vi "Documentation.vi"   [LabVIEW 2019, in "Instrument.Framework-Template.lvclass"]
uses:
  Instrument.Framework-Template.lvclass
  9169cc93-ed84-4232-9f90-6ee16c7bb454.vi
  de41cf0e-ff2b-4a51-852c-55dbec0e345b.vi
  9169cc93-ed84-4232-9f90-6ee16c7bb454.vi/3bc1a7ce-2052-4bb6-955b-7b4bb15f1b3f.vi
  de41cf0e-ff2b-4a51-852c-55dbec0e345b.vi/21da6090-1418-40bf-b1d0-aaaa039838a5.vi
  9169cc93-ed84-4232-9f90-6ee16c7bb454.vi/3bc1a7ce-2052-4bb6-955b-7b4bb15f1b3f.vi/186c7484-df9a-4054-807c-655d760e15c8.vi
  SMOs/Instrument/API/Send and Receive.vi
  9169cc93-ed84-4232-9f90-6ee16c7bb454.vi/3bc1a7ce-2052-4bb6-955b-7b4bb15f1b3f.vi/d68663b6-9a59-49ac-8a3e-6c41418329a1.vi
  SMOs/Instrument/Private/Get Client Type.vi
  de41cf0e-ff2b-4a51-852c-55dbec0e345b.vi/21da6090-1418-40bf-b1d0-aaaa039838a5.vi/9c6ae891-6b7b-494d-b8a3-540145664cba.vi
  de41cf0e-ff2b-4a51-852c-55dbec0e345b.vi/21da6090-1418-40bf-b1d0-aaaa039838a5.vi/557a546d-74cb-4577-b055-fbd1aae73a04.vi
  9169cc93-ed84-4232-9f90-6ee16c7bb454.vi/3bc1a7ce-2052-4bb6-955b-7b4bb15f1b3f.vi/186c7484-df9a-4054-807c-655d760e15c8.vi/d1b53759-cdad-4b30-913c-d0af3a047282.vi
  9169cc93-ed84-4232-9f90-6ee16c7bb454.vi/3bc1a7ce-2052-4bb6-955b-7b4bb15f1b3f.vi/186c7484-df9a-4054-807c-655d760e15c8.vi/7fe9f392-2cd1-45ec-9a03-6ef05e8253b6.vi
  9169cc93-ed84-4232-9f90-6ee16c7bb454.vi/3bc1a7ce-2052-4bb6-955b-7b4bb15f1b3f.vi/d68663b6-9a59-49ac-8a3e-6c41418329a1.vi/8fac68c8-b375-4435-9af1-ae7d05afa959.vi
  9169cc93-ed84-4232-9f90-6ee16c7bb454.vi/3bc1a7ce-2052-4bb6-955b-7b4bb15f1b3f.vi/d68663b6-9a59-49ac-8a3e-6c41418329a1.vi/1362d31b-bfc4-4d78-893d-5589c90f5b2b.vi
  de41cf0e-ff2b-4a51-852c-55dbec0e345b.vi/21da6090-1418-40bf-b1d0-aaaa039838a5.vi/9c6ae891-6b7b-494d-b8a3-540145664cba.vi/19fa3c45-0d16-4bb0-b2ad-138c00be1b64.vi
  de41cf0e-ff2b-4a51-852c-55dbec0e345b.vi/21da6090-1418-40bf-b1d0-aaaa039838a5.vi/9c6ae891-6b7b-494d-b8a3-540145664cba.vi/55c769c2-5611-4ccb-aecc-8b538907d375.vi
  de41cf0e-ff2b-4a51-852c-55dbec0e345b.vi/21da6090-1418-40bf-b1d0-aaaa039838a5.vi/557a546d-74cb-4577-b055-fbd1aae73a04.vi/b0531fe4-9e29-4687-baa2-aadea3dcdf03.vi
  de41cf0e-ff2b-4a51-852c-55dbec0e345b.vi/21da6090-1418-40bf-b1d0-aaaa039838a5.vi/557a546d-74cb-4577-b055-fbd1aae73a04.vi/d5c1aeff-1834-4139-868c-d1c2b7ad11df.vi
  9169cc93-ed84-4232-9f90-6ee16c7bb454.vi/3bc1a7ce-2052-4bb6-955b-7b4bb15f1b3f.vi/d68663b6-9a59-49ac-8a3e-6c41418329a1.vi/8fac68c8-b375-4435-9af1-ae7d05afa959.vi/29d737dc-f0a6-4278-8ea1-10f2043af5e9.vi
  9169cc93-ed84-4232-9f90-6ee16c7bb454.vi/3bc1a7ce-2052-4bb6-955b-7b4bb15f1b3f.vi/d68663b6-9a59-49ac-8a3e-6c41418329a1.vi/8fac68c8-b375-4435-9af1-ae7d05afa959.vi/10a74567-eb18-4897-8559-1a35f16d5028.vi
  de41cf0e-ff2b-4a51-852c-55dbec0e345b.vi/21da6090-1418-40bf-b1d0-aaaa039838a5.vi/557a546d-74cb-4577-b055-fbd1aae73a04.vi/b0531fe4-9e29-4687-baa2-aadea3dcdf03.vi/aeda4fc1-3546-460b-8fa5-afdc0bea1e87.vi
  de41cf0e-ff2b-4a51-852c-55dbec0e345b.vi/21da6090-1418-40bf-b1d0-aaaa039838a5.vi/557a546d-74cb-4577-b055-fbd1aae73a04.vi/b0531fe4-9e29-4687-baa2-aadea3dcdf03.vi/ed5f9993-61e6-48eb-895f-b725d41d8077.vi
  SMOs/Instrument/Private/Get RC Connection Status.vi
  SMOs/Instrument/API/Enum to String.vi
  SMOs/RemoteControl/API/Send and Receive.vi
  <vilib>/Utility/Data Type/Get Type Information.vi
  <vilib>/JDP Science/JSONtext/JSON text to Variant.vi
  SMOs/Instrument/API/Instrument.GetPublicEvents.vi
  <vilib>/JDP Science/JSONtext/Variant to JSON Text.vi
  <vilib>/National Instruments/GUID Generator/Guid Generator.vi
  SMOs/Instrument/Private/Instrument.MessageFromProcess.EventStructure.vi
  SMOs/Instrument/Instrument.lvclass
  <vilib>/JKI/JKI SMO/SMO/SMO.lvclass
  Typedefs/Instrument.Framework-Template.Commands--Enum.ctl
  Typedefs/Instrument.Framework-Template.getAll--Cluster.ctl
  Typedefs/Instrument.Framework-Template.Configuration--Cluster.ctl
  <vilib>/JDP Science/JSONtext/LVClass Serializer/JSONtext LVClass Serializer.lvclass
  Instrument UI.Framework-Template/Instrument UI.Framework-Template.lvclass
  Instrument UI.Framework-Template/Instrument UI.Framework-Template.UI--Cluster.ctl
  SMOs/Instrument UI/Instrument UI.lvclass
  <vilib>/JKI/JKI SMO/SMO.UI/SMO.UI.lvclass
  C:/Program Files (x86)/National Instruments/LabVIEW 2019/vi.lib/JKI/JKI SMO/SMO/SMO.lvclass
  C:/Users/patrick/Documents/GitHub/Instrument-Framework/lvsrc/SMOs/Instrument/Instrument.lvclass
  C:/Users/patrick/Documents/GitHub/Instrument-Framework/lvsrc/SMOs/Instrument UI/Instrument UI.lvclass
  C:/Program Files (x86)/National Instruments/LabVIEW 2019/vi.lib/JKI/JKI SMO/SMO.UI/SMO.UI.lvclass
types:
  T1 = typedef "Instrument.Framework-Template.lvclass/Instrument.Framework-Template.Configuration--Cluster.ctl" = cluster{"Example Setting 1":dbl, "Example Setting 2":dbl, "Example Setting 3":string}
  T2 = typedef "Instrument.Framework-Template.lvclass/Instrument.Framework-Template.getAll--Cluster.ctl" = cluster{"Levy 1":dbl, "Logger SMO":dbl, "SMO Boolean":bool, "SMO String":string}
  T3 = typedef "Instrument.Framework-Template.lvclass/Instrument.Framework-Template.Commands--Enum.ctl" = enum16{"Do Something"}
  T4 = typedef "Instrument UI.Framework-Template.lvclass/Instrument UI.Framework-Template.UI--Cluster.ctl" = cluster{"Parameter":dbl, "Parameter 2":string}
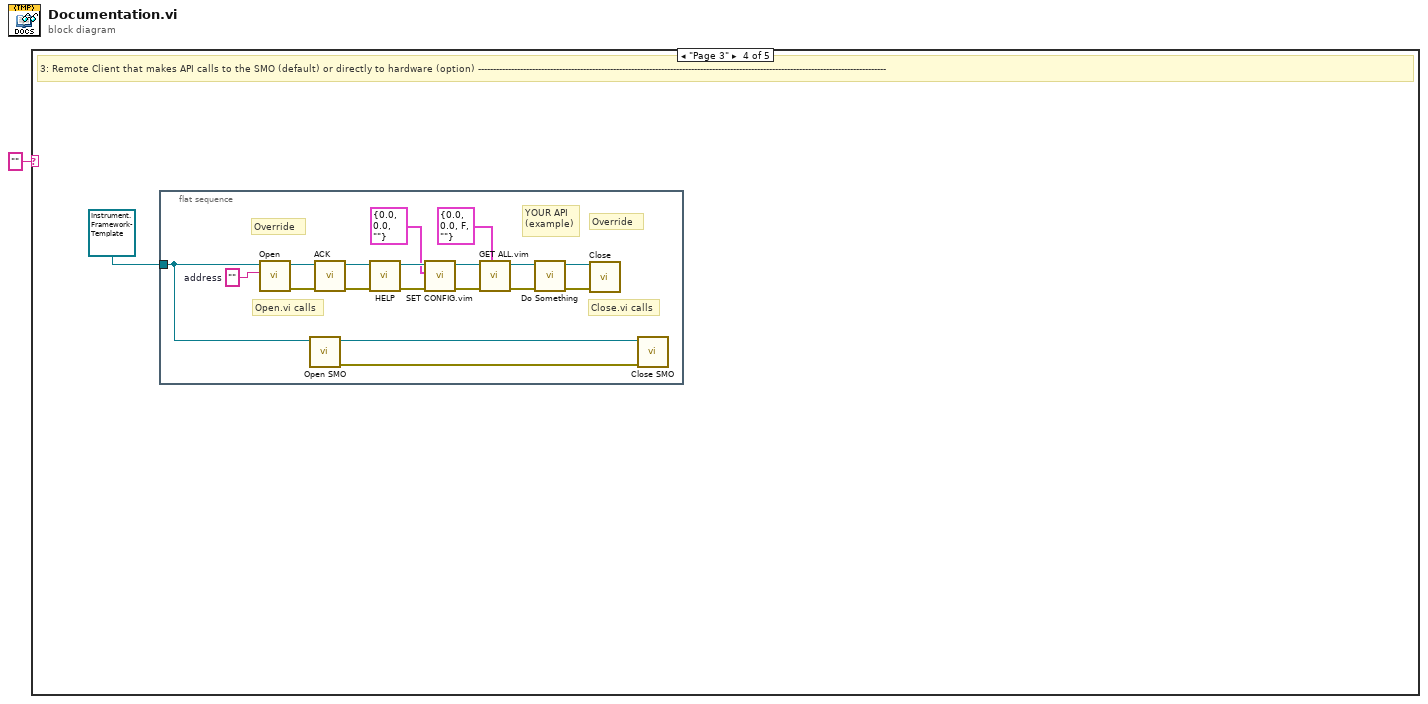
[diagram p0: block diagram]
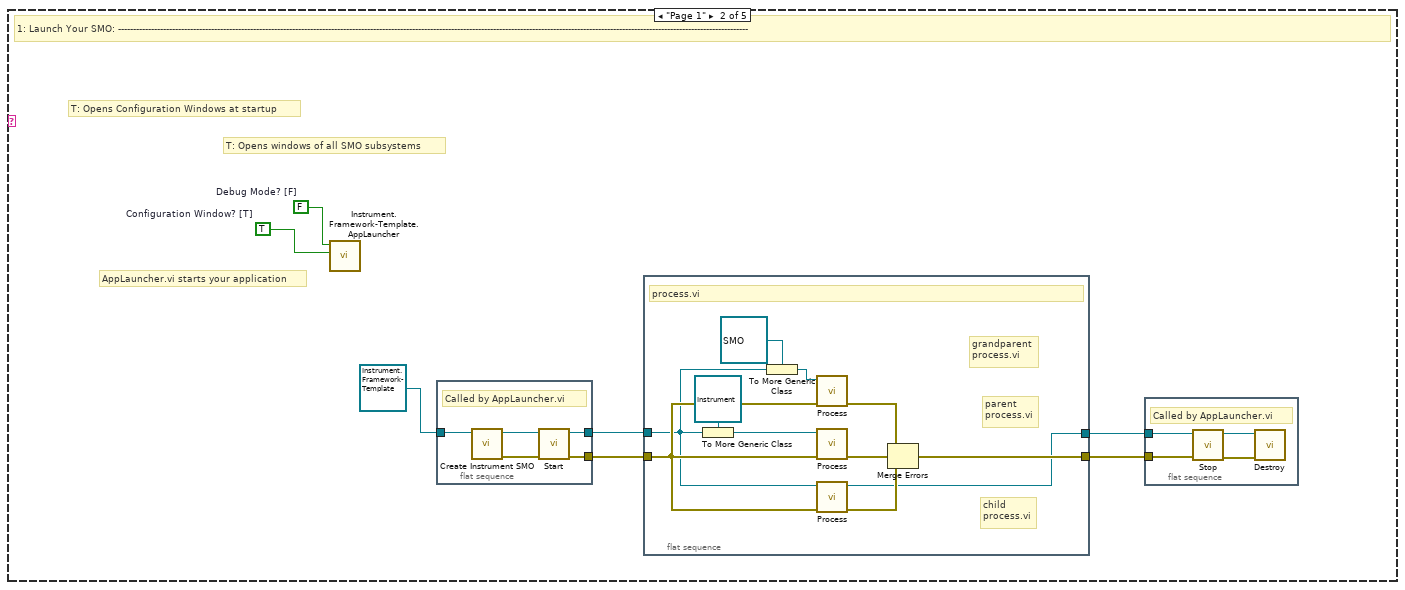
[diagram p3: hidden frame]
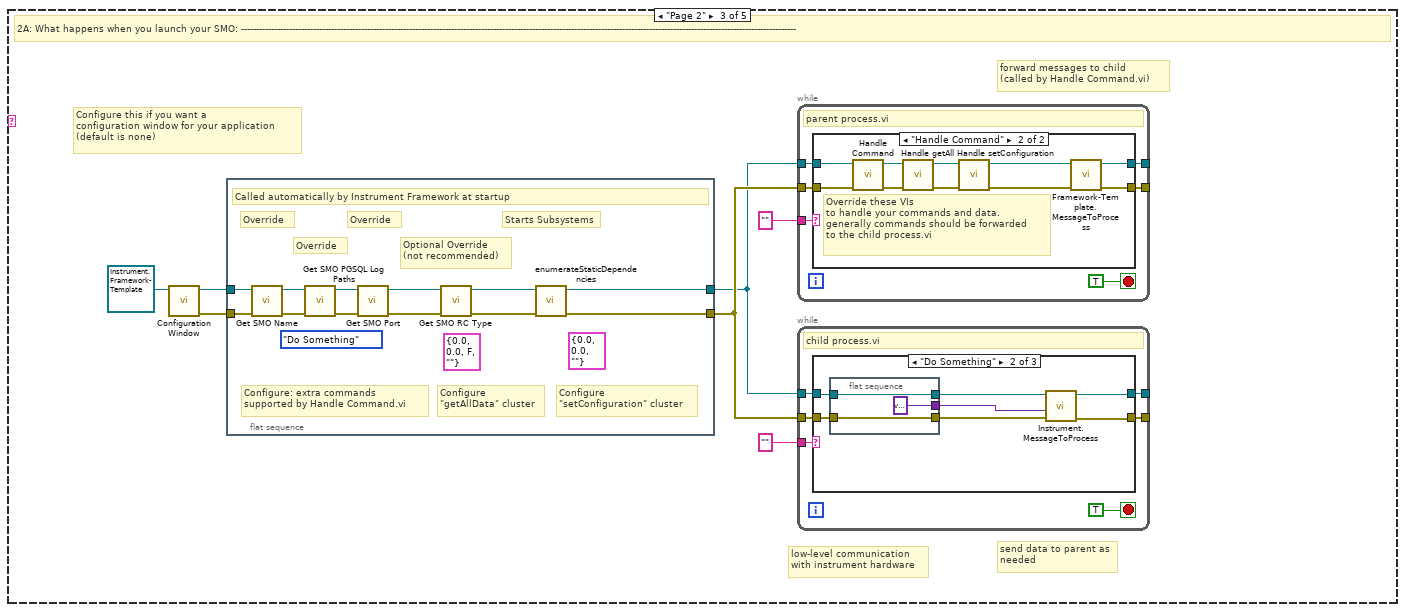
[diagram p4: hidden frame]
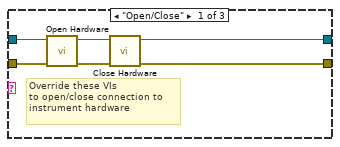
[diagram p5: hidden frame]
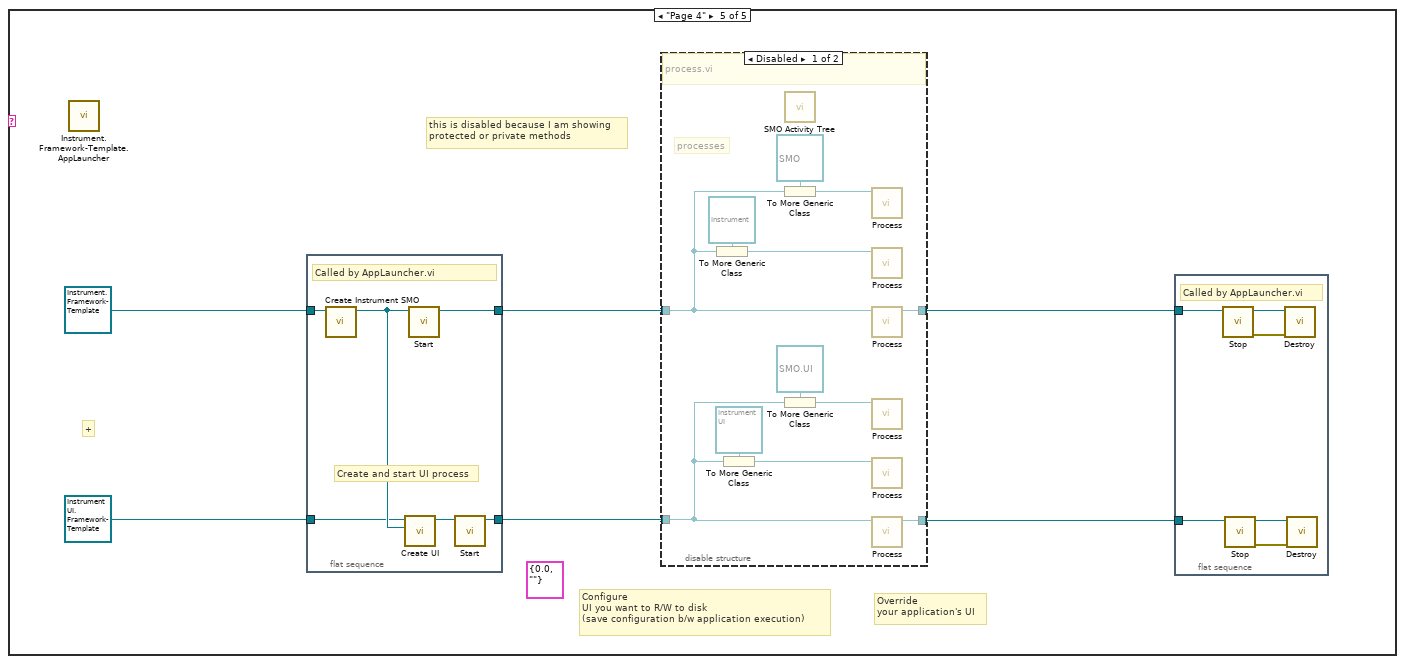
[diagram p8: hidden frame]
diagram:
  n1 = case shown="\"Page 3\"" "" {
    frame Default {
    }
    frame "Page 1" {
      w7 = TRUE  # Configuration Window? [T]
      w8 = FALSE  # Debug Mode? [F]
      # "AppLauncher.vi starts your application"
      # "T: Opens windows of all SMO subsystems"
      # "T: Opens Configuration Windows at startup"
      # "1: Launch Your SMO: ------------------------------------------------------------------------------------------------------------------------------------------------------------------------------------------------------------------"
      n2 = call "Instrument.Framework-Template.AppLauncher.vi"("Config Window"=w7, "Debug Mode"=w8) -> ()  [unwired: 9 in, 1 out]
      n3 = flat-sequence {
        tunnel: [w26] -> w3
        tunnel: [w25] -> w5
        tunnel: refnum<class "Instrument.Framework-Template.lvclass"> refnum ("Instrument.Template.lvclass") -> [w24]
        frame #0 {
          # "Called by AppLauncher.vi"
          n4 = call-dynamic "Create Instrument SMO.vi"("Instrument in"=w24) -> ("error out"=w27:errorcluster, "Instrument out"=w28:refnum<class "Instrument.Framework-Template.lvclass">)  [unwired: 9 in]
          n5 = call <vilib>:"Start.vi"("error in (no error)"=w27, "SMO"=w28) -> ("error out"=w25:errorcluster, "SMO out"=w26:refnum<class "Instrument.Framework-Template.lvclass">)  [unwired: 8 in]
        }
      }
      n6 = flat-sequence {
        tunnel: [w19] -> w6
        tunnel: w5 -> [w17]
        tunnel: [w11] -> w4
        tunnel: w3 -> [w10]
        frame #0 {
          # "child\nprocess.vi"
          # "grandparent\nprocess.vi"
          # "parent\nprocess.vi"
          # "process.vi"
          n7 = To More Generic Class(target class=refnum<class "Instrument.lvclass"> refnum ("Instrument"), reference=w10) -> (generic class reference=w16:refnum<class "Instrument.lvclass">)
          n8 = To More Generic Class(target class=refnum<class "SMO.lvclass"> refnum ("SMO"), reference=w10) -> (generic class reference=w18:refnum<class "SMO.lvclass">)
          n9 = call-dynamic "Process.vi"("error in"=w17, "SMO"=w18) -> ("error out"=w12:errorcluster)  [unwired: 8 in, 1 out]
          n10 = call-dynamic "Process.vi"("error in"=w17, "Instrument"=w16) -> ("error out"=w14:errorcluster)  [unwired: 8 in, 1 out]
          n11 = call-dynamic "Process.vi"("error in"=w17, "Framework-Template"=w10) -> ("error out"=w13:errorcluster, "Framework-Template out"=w11:refnum<class "Instrument.Framework-Template.lvclass">)  [unwired: 8 in]
          n12 = Merge Errors(w12, w14, w13) -> (w19:errorcluster)
        }
      }
      n13 = flat-sequence {
        tunnel: w4 -> [w21]
        tunnel: w6 -> [w20]
        frame #0 {
          # "Called by AppLauncher.vi"
          n14 = call <vilib>:"Stop.vi"("error in (no error)"=w20, "SMO"=w21) -> ("error out"=w23:errorcluster, "SMO out"=w22:refnum<class "Instrument.Framework-Template.lvclass">)  [unwired: 8 in]
          n15 = call <vilib>:"Destroy.vi"("error in (no error)"=w23, "SMO"=w22) -> ()  [unwired: 9 in, 1 out]
        }
      }
    }
    frame "Page 2" {
      # "forward messages to child\n(called by Handle Command.vi)"
      # "low-level communication\nwith instrument hardware"
      # "send data to parent as\nneeded"
      # "Configure this if you want a\nconfiguration window for your application\n(default is none)"
      # "2A: What happens when you launch your SMO: -----------------------------------------------------------------------------------------------------------------------------------------------------------------------------------------"
      n16 = call-dynamic "Configuration Window.vi"("Example Instrument in"=refnum<class "Instrument.Framework-Template.lvclass"> refnum ("Instrument.Template.lvclass")) -> ("error out"=w33:errorcluster, "Example Instrument out"=w35:refnum<class "Instrument.Framework-Template.lvclass">)  [unwired: 9 in]
      n17 = flat-sequence {
        tunnel: w35 -> [w85]
        tunnel: w33 -> [w80]
        tunnel: [w79] -> w30
        tunnel: [w78] -> w29
        frame #0 {
          (unwired) T1 {"Example Setting 1"=0.0, "Example Setting 2"=0.0, "Example Setting 3"=""} ("Configuration")
          (unwired) T2 {"Levy 1"=0.0, "Logger SMO"=0.0, "SMO Boolean"=FALSE, "SMO String"=""} ("getAll")
          (unwired) Instrument.Framework-Template.Commands--Enum."Do Something" ("Commands")
          # "Configure\n\"setConfiguration\" cluster"
          # "Configure\n\"getAllData\" cluster"
          # "Configure: extra commands\nsupported by Handle Command.vi"
          # "Starts Subsystems"
          # "Override"
          # "Override"
          # "Override"
          # "Optional Override\n(not recommended)"
          # "Called automatically by Instrument Framework at startup"
          n18 = call-dynamic "Get SMO Name.vi"("error in (no error)"=w80, "Example Instrument in"=w85) -> ("error out"=w83:errorcluster, "Example Instrument out"=w84:refnum<class "Instrument.Framework-Template.lvclass">)  [unwired: 7 in, 1 out]
          n19 = call-dynamic "Get SMO PGSQL Log Paths.vi"("error in (no error)"=w83, "Example in"=w84) -> ("error out"=w81:errorcluster, "Example out"=w82:refnum<class "Instrument.Framework-Template.lvclass">)  [unwired: 7 in, 1 out]
          n20 = call-dynamic "Get SMO Port.vi"("error in (no error)"=w81, "ExampleInstrument in"=w82) -> ("error out"=w86:errorcluster, "ExampleInstrument out"=w87:refnum<class "Instrument.Framework-Template.lvclass">)  [unwired: 7 in, 1 out]
          n21 = call-dynamic "Get SMO RC Type.vi"("error in (no error)"=w86, "ExampleInstrument in"=w87) -> ("error out"=w88:errorcluster, "ExampleInstrument out"=w89:refnum<class "Instrument.Framework-Template.lvclass">)  [unwired: 7 in, 1 out]
          n22 = call-dynamic "enumerateStaticDependencies.vi"("error in (no error)"=w88, "Instrument"=w89) -> ("error out"=w79:errorcluster, "Instrument out"=w78:refnum<class "Instrument.Framework-Template.lvclass">)  [unwired: 7 in, 1 out]
        }
      }
      n23 = while {
        tunnel: "" -> [w65]
        tunnel: w29 -> [w63]
        tunnel: [w62] -> _
        tunnel: w30 -> [w61]
        tunnel: [w60] -> _
        stop <- TRUE stop-if-true
        # "parent process.vi"
        n24 = case shown="\"Handle Command\"" w65 {
          tunnel: w63 -> [w67 w77]
          tunnel: [w67 w70] -> w62
          tunnel: w61 -> [w66 w76]
          tunnel: [w66 w69] -> w60
          frame Default {
          }
          frame "Handle Command" {
            # "Override these VIs\nto handle your commands and data.\ngenerally commands should be forwarded\nto the child process.vi"
            n25 = call-dynamic "Handle Command.vi"("error in (no error)"=w76, "Example Instrument in"=w77) -> ("error out"=w72:errorcluster, "Example Instrument out"=w75:refnum<class "Instrument.Framework-Template.lvclass">)  [unwired: 6 in, 2 out]
            n26 = call-dynamic "Handle getAll.vi"("error in (no error)"=w72, "Example Instrument in"=w75) -> ("error out"=w73:errorcluster, "Example Instrument out"=w74:refnum<class "Instrument.Framework-Template.lvclass">)  [unwired: 7 in, 1 out]
            n27 = call-dynamic "Handle setConfiguration.vi"("error in (no error)"=w73, "Instrument.Template in"=w74) -> ("error out"=w68:errorcluster, "Instrument.Template out"=w71:refnum<class "Instrument.Framework-Template.lvclass">)  [unwired: 8 in]
            n28 = call "Framework-Template.MessageToProcess.vi"("error in (no error)"=w68, "Framework-Template in"=w71) -> ("error out"=w69:errorcluster, "Framework-Template out"=w70:refnum<class "Instrument.Framework-Template.lvclass">)  [unwired: 8 in]
          }
        }
      }
      n29 = while {
        tunnel: "" -> [w41]
        tunnel: w29 -> [w39]
        tunnel: [w38] -> _
        tunnel: w30 -> [w37]
        tunnel: [w36] -> _
        stop <- TRUE stop-if-true
        # "child process.vi"
        n30 = case shown="\"Do Something\"" w41 {
          tunnel: w39 -> [w44 w50 w59]
          tunnel: [w43 w54 w59] -> w38
          tunnel: w37 -> [w47 w52 w58]
          tunnel: [w42 w53 w58] -> w36
          frame "Open/Close" {
            # "Override these VIs\nto open/close connection to\ninstrument hardware"
            n31 = call-dynamic "Open Hardware.vi"("error in (no error)"=w47, "Instrument.Template in"=w44) -> ("error out"=w46:errorcluster, "Instrument.Template out"=w45:refnum<class "Instrument.Framework-Template.lvclass">)  [unwired: 8 in]
            n32 = call-dynamic "Close Hardware.vi"("error in (no error)"=w46, "Instrument.Template in"=w45) -> ("error out"=w42:errorcluster, "Instrument.Template out"=w43:refnum<class "Instrument.Framework-Template.lvclass">)  [unwired: 8 in]
          }
          frame "Do Something" {
            n33 = flat-sequence {
              tunnel: w52 -> [w57]
              tunnel: [w57] -> w51
              tunnel: w50 -> [w56]
              tunnel: [w56] -> w49
              tunnel: [variant ("Data")] -> w48
              frame #0 {
              }
            }
            n34 = call "Instrument.MessageToProcess.vi"("error in (no error)"=w51, "Data"=w48, "Instrument"=w49) -> ("error out"=w53:errorcluster, "Instrument out"=w54:refnum<class "Instrument.Framework-Template.lvclass">)  [unwired: 7 in]
          }
          frame Default {
          }
        }
      }
    }
    frame "Page 3" {
      # "3: Remote Client that makes API calls to the SMO (default) or directly to hardware (option) ----------------------------------------------------------------------------------------------------------------------------------------"
      n35 = flat-sequence {
        tunnel: refnum<class "Instrument.Framework-Template.lvclass"> refnum ("Instrument.Template.lvclass") -> [w91]
        frame #0 {
          w94 = ""  # address
          # "Close.vi calls"
          # "Open.vi calls"
          # "YOUR API\n(example)"
          # "Override"
          # "Override"
          n36 = call-dynamic "Open.vi"("address"=w94, "Instrument.Template in"=w91) -> ("error out"=w108:errorcluster, "Instrument.Template out"=w107:refnum<class "Instrument.Framework-Template.lvclass">)  [unwired: 8 in]
          n37 = call "Open SMO.vi"("Instrument in"=w91) -> ("error out"=w92:errorcluster, "Instrument out"=w93:refnum<class "Instrument.Framework-Template.lvclass">)  [unwired: 9 in]
          n38 = call "ACK.vi"("error in (no error)"=w108, "Instrument in"=w107) -> ("error out"=w106:errorcluster, "Instrument out"=w105:refnum<class "Instrument.Framework-Template.lvclass">)  [unwired: 7 in, 1 out]
          n39 = call "HELP.vi"("error in (no error)"=w106, "Instrument in"=w105) -> ("error out"=w100:errorcluster, "Instrument in"=w101:refnum<class "Instrument.Framework-Template.lvclass">)  [unwired: 7 in, 1 out]
          n40 = call "SET CONFIG.vim"("error in (no error)"=w100, "Configuration"=T1 {"Example Setting 1"=0.0, "Example Setting 2"=0.0, "Example Setting 3"=""}, "Instrument in"=w101) -> ("error out"=w95:errorcluster, "Instrument out"=w98:refnum<class "Instrument.Framework-Template.lvclass">)  [unwired: 7 in]
          n41 = call "GET ALL.vim"("type"=T2 {"Levy 1"=0.0, "Logger SMO"=0.0, "SMO Boolean"=FALSE, "SMO String"=""} ("getAll"), "error in (no error)"=w95, "Instrument in"=w98) -> ("error out"=w96:errorcluster, "Instrument out"=w97:refnum<class "Instrument.Framework-Template.lvclass">)  [unwired: 6 in, 1 out]
          n42 = call-dynamic "Do Something.vi"("error in (no error)"=w96, "Example in"=w97) -> ("error out"=w103:errorcluster, "Example out"=w104:refnum<class "Instrument.Framework-Template.lvclass">)  [unwired: 8 in]
          n43 = call-dynamic "Close.vi"("error in (no error)"=w103, "Instrument.Template in"=w104) -> ()  [unwired: 8 in, 2 out]
          n44 = call "Close SMO.vi"("error in (no error)"=w92, "Instrument in"=w93) -> ()  [unwired: 8 in, 2 out]
        }
      }
    }
    frame "Page 4" {
      (unwired) T4 {"Parameter"=0.0, "Parameter 2"=""} ("UI")
      # "this is disabled because I am showing\nprotected or private methods"
      # "Configure\nUI you want to R/W to disk\n(save configuration b/w application execution)"
      # "Override\nyour application's UI"
      # "+"
      n45 = call "Instrument.Framework-Template.AppLauncher.vi"() -> ()  [unwired: 11 in, 1 out]
      n46 = flat-sequence {
        tunnel: [w126] -> w112
        tunnel: refnum<class "Instrument.Framework-Template.lvclass"> refnum ("Instrument.Template.lvclass") -> [w125]
        tunnel: refnum<class "Instrument UI.Framework-Template.lvclass"> refnum ("Instrument UI.Template.lvclass") -> [w123]
        tunnel: [w121] -> w110
        frame #0 {
          # "Create and start UI process"
          # "Called by AppLauncher.vi"
          n47 = call-dynamic "Create Instrument SMO.vi"("Instrument in"=w125) -> ("Instrument out"=w124:refnum<class "Instrument.Framework-Template.lvclass">)  [unwired: 9 in, 1 out]
          n48 = call "Create UI.vi"("Instrument in"=w124, "Instrument UI"=w123) -> ("Instrument UI out"=w122:refnum<class "Instrument UI.Framework-Template.lvclass">)  [unwired: 8 in, 1 out]
          n49 = call <vilib>:"Start.vi"("SMO"=w124) -> ("SMO out"=w126:refnum<class "Instrument.Framework-Template.lvclass">)  [unwired: 9 in, 1 out]
          n50 = call <vilib>:"Start.vi"("SMO"=w122) -> ("SMO out"=w121:refnum<class "Instrument UI.Framework-Template.lvclass">)  [unwired: 9 in, 1 out]
        }
      }
      n51 = disable-structure shown="Disabled" {
        disable-tunnel: [w138 w140] -> w113
        disable-tunnel: w112 -> [w137 w140]
        disable-tunnel: w110 -> [w136 w139]
        disable-tunnel: [w135 w139] -> w109
        frame Disabled {
          # "processes"
          # "process.vi"
          n52 = To More Generic Class(target class=refnum<class "Instrument.lvclass"> refnum ("Instrument"), reference=w137) -> (generic class reference=w133:refnum<class "Instrument.lvclass">)
          n53 = To More Generic Class(target class=refnum<class "Instrument UI.lvclass"> refnum ("Instrument UI"), reference=w136) -> (generic class reference=w129:refnum<class "Instrument UI.lvclass">)
          n54 = call <vilib>:"SMO Activity Tree.vi"() -> ()  [unwired: 12 in]
          n55 = To More Generic Class(target class=refnum<class "SMO.lvclass"> refnum ("SMO"), reference=w137) -> (generic class reference=w134:refnum<class "SMO.lvclass">)
          n56 = To More Generic Class(target class=refnum<class "SMO.UI.lvclass"> refnum ("SMO.UI"), reference=w136) -> (generic class reference=w127:refnum<class "SMO.UI.lvclass">)
          n57 = call-dynamic "Process.vi"("SMO"=w134) -> ()  [unwired: 9 in, 2 out]
          n58 = call-dynamic "Process.vi"("Instrument"=w133) -> ()  [unwired: 9 in, 2 out]
          n59 = call-dynamic "Process.vi"("Framework-Template"=w137) -> ("Framework-Template out"=w138:refnum<class "Instrument.Framework-Template.lvclass">)  [unwired: 9 in, 1 out]
          n60 = call-dynamic "Process.vi"("SMO.UI"=w127) -> ()  [unwired: 9 in, 2 out]
          n61 = call-dynamic "Process.vi"("Instrument UI in"=w129) -> ()  [unwired: 9 in, 2 out]
          n62 = call-dynamic "Process.vi"("Example Instrument UI"=w136) -> ("Example Instrument UI out"=w135:refnum<class "Instrument UI.Framework-Template.lvclass">)  [unwired: 9 in, 1 out]
        }
        frame Enabled {
        }
      }
      n63 = flat-sequence {
        tunnel: w113 -> [w118]
        tunnel: w109 -> [w116]
        frame #0 {
          # "Called by AppLauncher.vi"
          n64 = call <vilib>:"Stop.vi"("SMO"=w118) -> ("error out"=w120:errorcluster, "SMO out"=w119:refnum<class "Instrument.Framework-Template.lvclass">)  [unwired: 9 in]
          n65 = call <vilib>:"Stop.vi"("SMO"=w116) -> ("error out"=w117:errorcluster, "SMO out"=w115:refnum<class "Instrument UI.Framework-Template.lvclass">)  [unwired: 9 in]
          n66 = call <vilib>:"Destroy.vi"("error in (no error)"=w120, "SMO"=w119) -> ()  [unwired: 9 in, 1 out]
          n67 = call <vilib>:"Destroy.vi"("error in (no error)"=w117, "SMO"=w115) -> ()  [unwired: 9 in, 1 out]
        }
      }
    }
  }
